vi "get_Vtop_from_Efield_and_Vbot_2024lv.vi"(8 "V_bottom (V)":dbl format="%#_13g", 9 "Efield (V/nm)":dbl format="%#_13g", 10 "d_bottom (nm)":dbl format="%#_13g", 11 "d_top (nm)":dbl format="%#_13g") -> (2 "V_top (V)":dbl)   [LabVIEW 2024]
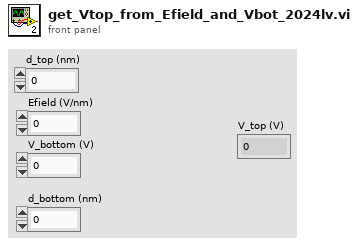
[diagram p1: front panel]
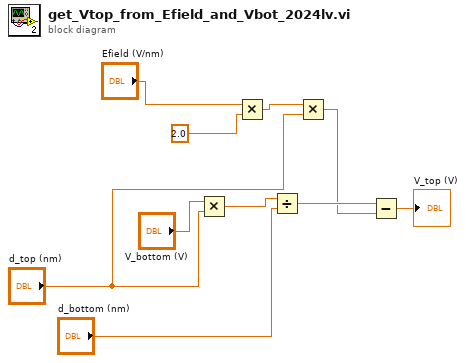
[diagram p0: block diagram]
diagram:
  n1 = Multiply(x="V_bottom (V)", y="d_top (nm)") -> (x*y=w9:dbl)
  n2 = Multiply(x="Efield (V/nm)", y=2.0) -> (x*y=w5:dbl)
  n3 = Divide(x=w9, y="d_bottom (nm)") -> (x/y=w3:dbl)
  n4 = Multiply(x=w5, y="d_top (nm)") -> (x*y=w2:dbl)
  n5 = Subtract(x=w3, y=w2) -> (x-y=→"V_top (V)":dbl)
